vi "NF WF1973_74 sample output.vi"(0 "VISAsession":refnum<visa-resource-name>, 1 "Ch?(Ch1)":bool, 2 "OUTPUT?(OFF)":bool, 5 "Select Function(Sine)":i32(ring)=2 items=["DC", "Noise", "Sinusoid", "Square", "Pulse", "Ramp", "USine", "CSine", "CFCSine", "ACSine", "SSine", "MCSine", "ONPSine", "OFPSine", "CONSine", "COFSine", "Gaussian", "Lorents", "Haversine", "HSPulse", "TPulse", "Sinc", "ERise", "EFall", "Solstep", "Doscillation", "OSurge", "PSurge", "TOffset", "HSEPulse", "BRRamp", "USER"], 7 "Frequency(1)":dbl=1.0 format="%.8f", 9 "Units(Hz)":u16(ring)=2 items=["Mega(M)", "Kilo(k)", "Hz", "Micro(u)", "Nano(n)"], 11 "error in (no error)":errorcluster caption="Error IN", 12 "Amplitude(1)":dbl=1.0 format="%.3f", 13 "Units(Vpp)":u16(ring) items=["Vpp", "Vpk", "Vrms", "dBv", "dBm", "USER", "mVpp", "mVpk", "mVrms"]) -> (4 "CopyVISAsession":refnum<visa-resource-name>, 15 "error out":errorcluster caption="Error OUT")   [LabVIEW 2010]
panel:
  # "WF1973/1974 OUTPUT SET VI"
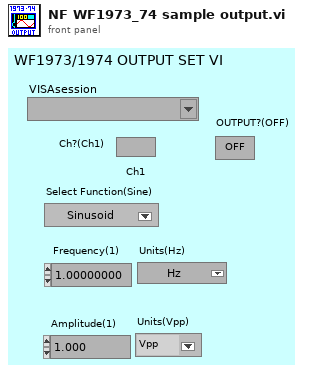
[diagram p1: front panel]
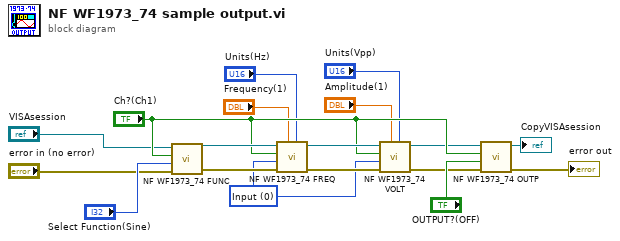
[diagram p0: block diagram]
diagram:
  w10 = u16 0 items=["Input", "Minimum", "Maximum"] ("Frequency type(Input)")
  n1 = call <instrlib>:"NF WF1973_74 FUNC.vi"("error in (no error)"="error in (no error)", "Select Function(Sin)"="Select Function(Sine)", "Ch?(Ch1)"="Ch?(Ch1)", "VISAsession"="VISAsession") -> ("error out"=w16:errorcluster, "CopyVISAsession"=w17:refnum<visa-resource-name>)  [unwired: 5 in, 1 out]
  n2 = call <instrlib>:"NF WF1973_74 FREQ.vi"("Units(Hz)"="Units(Hz)", "Frequency(1)"="Frequency(1)", "error in (no error)"=w16, "Set Frequency (Input)"=w10, "Ch(Ch1)"="Ch?(Ch1)", "VISAsession"=w17) -> ("error out"=w14:errorcluster, "CopyVISAsession"=w15:refnum<visa-resource-name>)  [unwired: 3 in, 1 out]
  n3 = call <instrlib>:"NF WF1973_74 VOLT.vi"("Units(Vpp)"="Units(Vpp)", "Amplitude(1)"="Amplitude(1)", "error in (no error)"=w14, "Set Amplitude(Input)"=w10, "Ch(Ch1)"="Ch?(Ch1)", "VISAsession"=w15) -> ("error out"=w5:errorcluster, "CopyVISAsession"=w4:refnum<visa-resource-name>)  [unwired: 3 in, 1 out]
  n4 = call <instrlib>:"NF WF1973_74 OUTP.vi"("error in (no error)"=w5, "Output(OFF)"="OUTPUT?(OFF)", "Ch(Ch1)"="Ch?(Ch1)", "VISAsession"=w4) -> ("error out"=→"error out":errorcluster, "CopyVISAsession"=→"CopyVISAsession":refnum<visa-resource-name>)  [unwired: 5 in, 1 out]
